vi "ENA_Initialize.vi"(8 "error in (no error)":errorcluster, 9 "Reset? (T: Yes)":bool=TRUE, 10 "ID Query? (T: Yes)":bool=TRUE, 11 "VISA resource name":refnum<visa-resource-name>) -> (0 "error out":errorcluster, 3 "VISA resource name out":refnum<visa-resource-name>)   [LabVIEW 2013]
doc: "Establishes communication with the instrument and optionally performs an instrument identification query and/or an instrument reset. It also places the instrument in a default state needed for other instrument driver operations. Therefore, call this VI before calling other instrument driver VIs for this instrument. Generally, you need to call the <B>Initialize VI</B> only once at the beginning of an application.\n\n<b>Note:</b>\nE5080A model support enabled by configuring the Emulation Mode \nSystem -> System Setting -> Code Emulation -> 5071"
uses:
  <vilib>/regexp/Match Regular Expression.xnode
panel:
  # "(c) 2005-2017 National Instruments.  ALL RIGHTS RESERVED."
  # "Note:\nE5080A model support enabled by configuring the Emulation Mode \nSystem -> System Setting -> Code Emulation -> 5071"
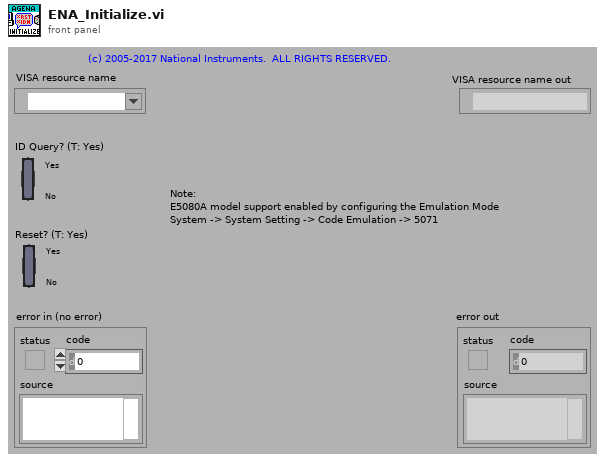
[diagram p1: front panel]
types:
  T1 = cluster{"Status":bool, "Code":i32, "Source (VI Name)":string}
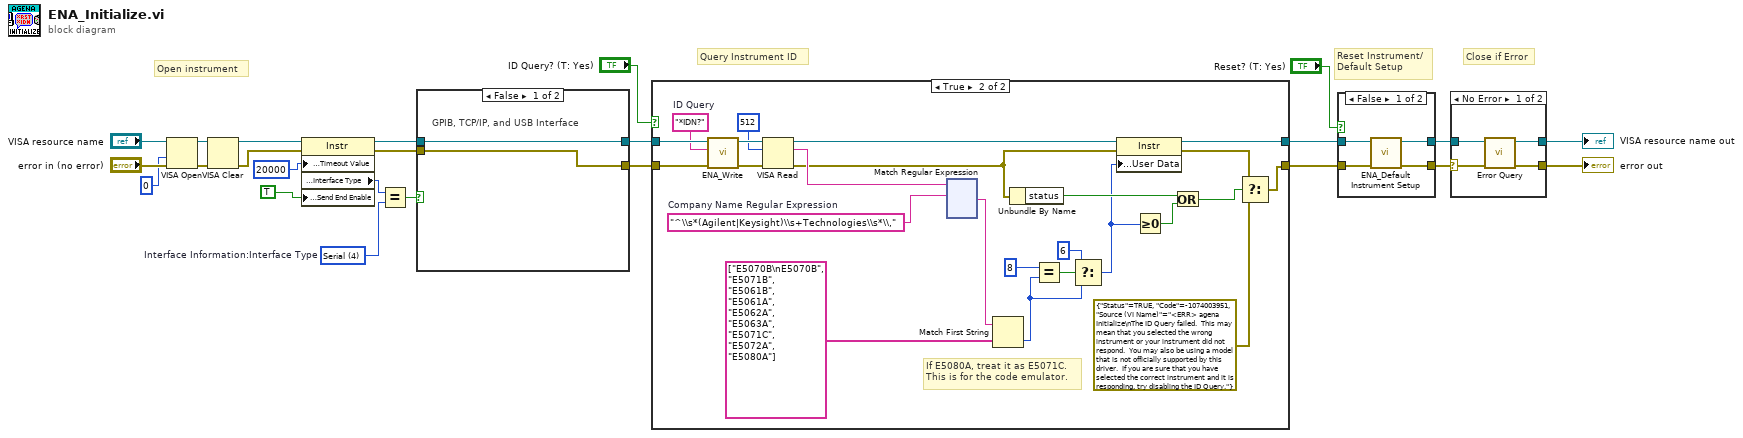
[diagram p0: block diagram]
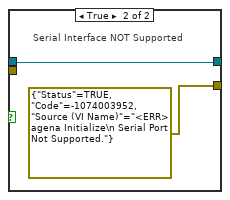
[diagram p2: hidden frame]
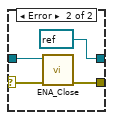
[diagram p3: hidden frame]
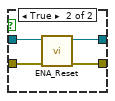
[diagram p4: hidden frame]
diagram:
  w13 = u16 4 items=["GPIB"=1, "VXI"=2, "GPIB-VXI"=3, "Serial"=4, "PXI"=5, "TCPIP"=6, "USB"=7]  # Interface Information:Interface Type
  # "Close if Error"
  # "Query Instrument ID"
  # "Reset Instrument/\nDefault Setup"
  # "Open instrument"
  n1 = VISA Open(access mode=u32 0, error in (no error)="error in (no error)", VISA resource name="VISA resource name") -> (VISA resource name=w3:refnum<visa-resource-name>, error out=w4:errorcluster)  [unwired: 2 in]
  n2 = VISA Clear(VISA resource name=w3, error in (no error)=w4) -> (VISA resource name out=w2:refnum<visa-resource-name>, error out=w1:errorcluster)
  n3 = property class="Instr"(reference=w2, error in=w1, "General Settings:Timeout Value"=u32 20000, "Message Based Settings:Send End Enable"=TRUE) -> (reference out=w16:refnum<visa-resource-name>, error out=w15:errorcluster, "Interface Information:Interface Type"=w18:u16)
  n4 = Equal?(x=w18, y=w13) -> (x = y?=w14:bool)
  n5 = case shown="False" w14 {
    tunnel: [w26 w28] -> w6
    tunnel: [w25 T1 {"Status"=TRUE, "Code"=-1074003952, "Source (VI Name)"="<ERR> agena Initialize\n Serial Port Not Supported."}] -> w5
    tunnel: w16 -> [w26 w28]
    tunnel: w15 -> [w25 _]
    frame False {
      # "GPIB, TCP/IP, and USB Interface"
    }
    frame True {
      # "Serial Interface NOT Supported"
    }
  }
  n6 = case shown="True" "ID Query? (T: Yes)" {
    tunnel: [w29 w54] -> w23
    tunnel: [w30 w40] -> w24
    tunnel: w6 -> [w30 w52]
    tunnel: w5 -> [w29 w53]
    frame False {
    }
    frame True {
      w37 = "^\\s*(Agilent|Keysight)\\s+Technologies\\s*\\,"  # Company Name Regular Expression
      w45 = "*IDN?"  # ID Query
      # "If E5080A, treat it as E5071C.\nThis is for the code emulator."
      n7 = call "ENA_Write.vi"("error in (no error)"=w53, "String ()"=w45, "VISA resource name"=w52) -> ("error out"=w49:errorcluster, "VISA resource name out"=w50:refnum<visa-resource-name>)  [unwired: 6 in, 1 out]
      n8 = VISA Read(VISA resource name=w50, byte count=u32 512, error in (no error)=w49) -> (VISA resource name out=w41:refnum<visa-resource-name>, read buffer=w43:string, error out=w39:errorcluster)  [unwired: 1 out]
      n9 = xnode "Match Regular Expression"("input string"=w43, "regular expression"=w37) -> ("after match"=w36:string)  [unwired: 4 in, 4 out]
      n10 = Match First String(2:string[] ["E5070B\nE5070B", "E5071B", "E5061B", "E5061A", "E5062A", "E5063A", "E5071C", "E5072A", "E5080A"] ("string array"), 3:w36) -> (0:w33:i32)  [unwired: 1 out]
      n11 = Unbundle By Name(w39) -> ("status"=w47:bool)
      n12 = Equal?(x=8, y=w33) -> (x = y?=w34:bool)
      n13 = Select(t=6, s=w34, f=w33) -> (s? t:f=w31:i32)
      n14 = property on="Property Node" class="Instr"(reference=w41, error in=w39, "General Settings:User Data"=w31) -> (reference out=w40:refnum<visa-resource-name>, error out=w38:errorcluster)
      n15 = Greater Or Equal To 0?(x=w31) -> (x >= 0?=w51:bool)
      n16 = Or(x=w47, y=w51) -> (x .or. y?=w48:bool)
      n17 = Select(t=w38, s=w48, f=T1 {"Status"=TRUE, "Code"=-1074003951, "Source (VI Name)"="<ERR> agena Initialize\nThe ID Query failed.  This may mean that you selected the wrong instrument or your instrument did not respond.  You may also be using a model that is not officially supported by this driver.  If you are sure that you have selected the correct instrument and it is responding, try disabling the ID Query."}) -> (s? t:f=w54:T1)
    }
  }
  n18 = case shown="False" "Reset? (T: Yes)" {
    tunnel: w23 -> [w171 w173]
    tunnel: [w170 w176] -> w8
    tunnel: w24 -> [w172 w174]
    tunnel: [w169 w175] -> w9
    frame False {
      n19 = call "ENA_Default Instrument Setup.vi"("error in (no error)"=w171, "VISA resource name"=w172) -> ("error out"=w170:errorcluster, "VISA resource name out"=w169:refnum<visa-resource-name>)  [unwired: 8 in]
    }
    frame True {
      n20 = call "ENA_Reset.vi"("error in (no error)"=w173, "VISA resource name"=w174) -> ("error out"=w176:errorcluster, "VISA resource name out"=w175:refnum<visa-resource-name>)  [unwired: 8 in]
    }
  }
  n21 = case shown="No Error" w8 {
    selector: w8 -> [w178 w182]
    tunnel: w9 -> [w177 w183]
    tunnel: [w180 refnum<visa-resource-name> refnum ("VISA resource name out")] -> w11
    tunnel: [w179 w184] -> w10
    frame No Error {
      n22 = call "Error Query.vi"("error in (no error)"=w178, "VISA resource name"=w177) -> ("error out"=w179:errorcluster, "VISA resource name out"=w180:refnum<visa-resource-name>)  [unwired: 6 in, 2 out]
    }
    frame Error {
      n23 = call "ENA_Close.vi"("error in (no error)"=w182, "VISA resource name"=w183) -> ("error out"=w184:errorcluster)  [unwired: 9 in]
    }
  }
  "VISA resource name out" <- w11
  "error out" <- w10
